vi "temp_FlpLib PI_Controller.vi"(0 "error":sgl format="%#_13g", 1 "reset? (F)":bool, 5 "enable bumpless transfer? (F)":bool, 7 "manual control":T5, 11 "state in":T2, 12 "gains":T3 {"proportional gain" step=0.125}, 13 "output range":T4={"output high (Inf)"=inf, "output low (-Inf)"=-inf}) -> (4 "output":sgl, 6 "error":sgl, 8 "actions":T1, 15 "state out":T2)   [LabVIEW 2016]
uses:
  <vilib>/rvi/Analysis/control/PID/Typedef/niFpgaPID_ManualControl.ctl
  <vilib>/rvi/Analysis/control/PID/Typedef/niFpgaPID_OutputRange.ctl
  <vilib>/rvi/Analysis/control/PID/Typedef/niFpgaPID_PIGains.ctl
  <vilib>/rvi/Analysis/control/PID/Typedef/niFpgaPID_PIState.ctl
  <vilib>/rvi/Analysis/control/PID/Typedef/niFpgaPID_PIActions.ctl
  <userlib>/_NI FLP Library/FPGA/outsideSCTL/FlpLib Multiply Shared Instance 0.vi
  <userlib>/_NI FLP Library/FPGA/outsideSCTL/FlpLib Add Shared Instance 0.vi
  <userlib>/_NI FLP Library/FPGA/outsideSCTL/FlpLib Subtract Shared Instance 0.vi
  <userlib>/_NI FLP Library/FPGA/outsideSCTL/FlpLib In Range and Coerce Shared Instance 0.vi
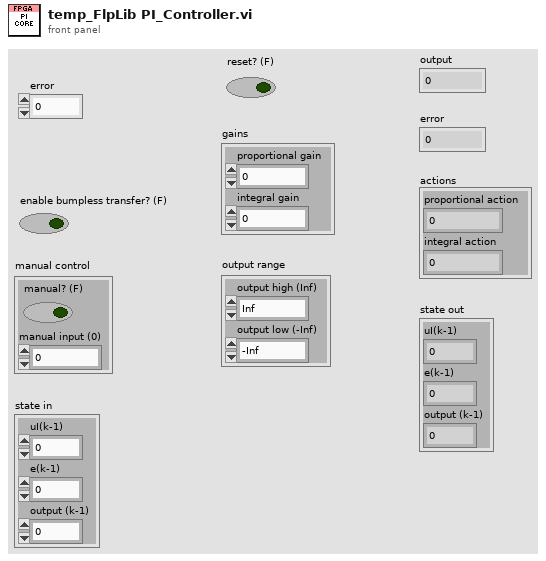
[diagram p1: front panel]
types:
  T1 = typedef "niFpgaPID_PIActions.ctl" = cluster{"proportional action":sgl, "integral action":sgl}
  T2 = typedef "niFpgaPID_PIState.ctl" = cluster{"uI(k-1)":sgl, "e(k-1)":sgl, "output (k-1)":sgl}
  T3 = typedef "niFpgaPID_PIGains.ctl" = cluster{"proportional gain":sgl, "integral gain":sgl}
  T4 = typedef "niFpgaPID_OutputRange.ctl" = cluster{"output high (Inf)":sgl, "output low (-Inf)":sgl}
  T5 = typedef "niFpgaPID_ManualControl.ctl" = cluster{"manual? (F)":bool, "manual input (0)":sgl}
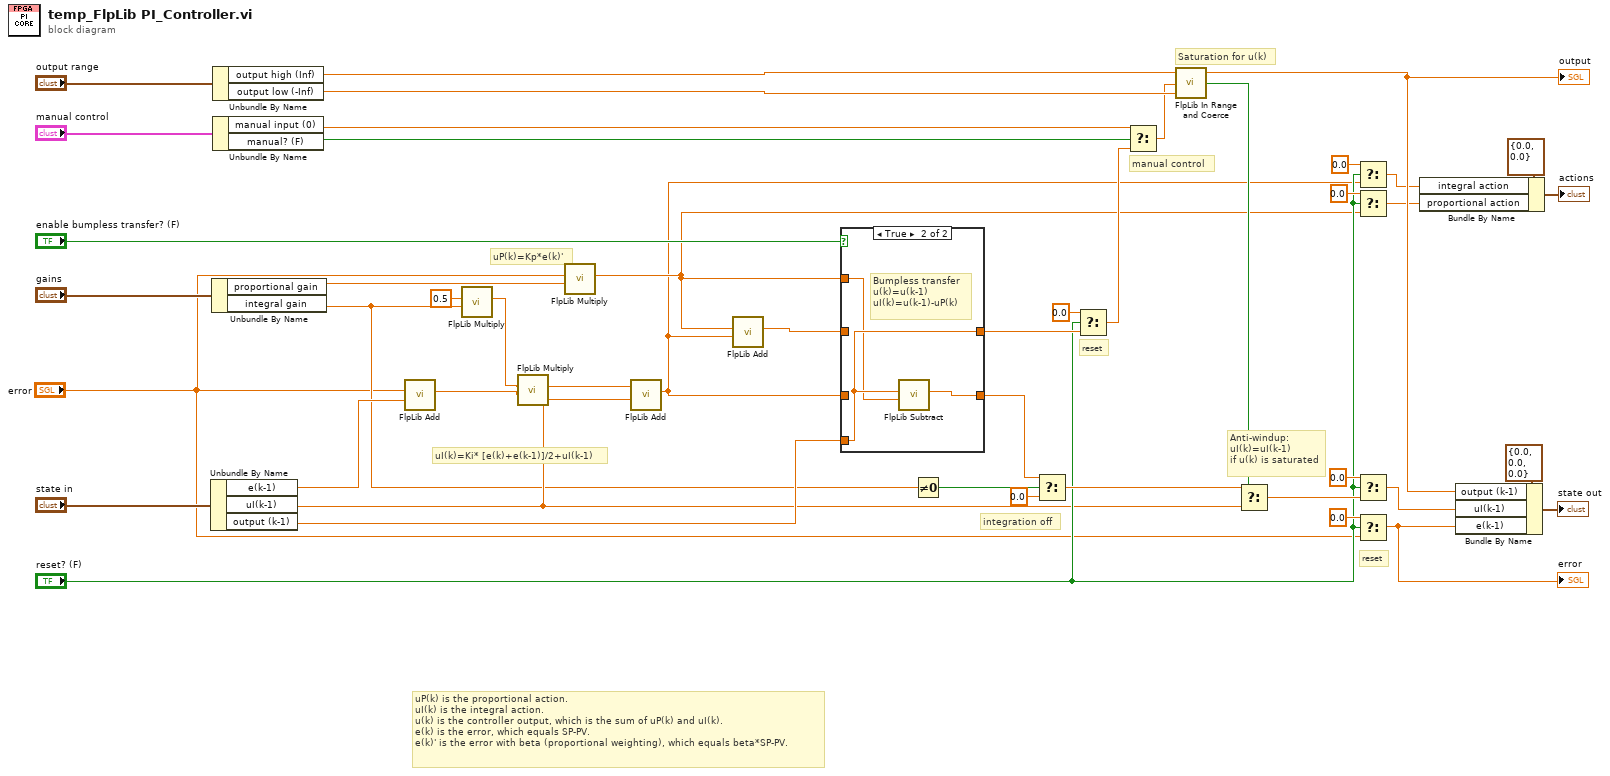
[diagram p0: block diagram]
diagram:
  # "uP(k) is the proportional action.\nuI(k) is the integral action.\nu(k) is the controller output, which is the sum of uP(k) and uI(k).\ne(k) is the error, which equals SP-PV.\ne(k)' is the error with beta (proportional weighting), which equals beta*SP-PV."
  # "integration off"
  # "reset"
  # "manual control"
  # "reset"
  # "Anti-windup:\nuI(k)=uI(k-1) \nif u(k) is saturated"
  # "Saturation for u(k)"
  # "uI(k)=Ki* [e(k)+e(k-1)]/2+uI(k-1)"
  # "uP(k)=Kp*e(k)'"
  n1 = Unbundle By Name("state in") -> ("e(k-1)"=w12:sgl, "uI(k-1)"=w11:sgl, "output (k-1)"=w39:sgl)
  n2 = Unbundle By Name("gains") -> ("proportional gain"=w8:sgl, "integral gain"=w3:sgl)
  n3 = Unbundle By Name("output range") -> ("output high (Inf)"=w27:sgl, "output low (-Inf)"=w26:sgl)
  n4 = Unbundle By Name("manual control") -> ("manual input (0)"=w36:sgl, "manual? (F)"=w35:bool)
  n5 = call-poly <userlib>:"FlpLib Add.vi"("y"=w12, "x"="error") -> ("x+y"=w10:sgl)  [unwired: 5 in]
  n6 = call-poly <userlib>:"FlpLib Multiply.vi"("y"=w3, "x"=sgl 0.5) -> ("x*y"=w4:sgl)  [unwired: 5 in]
  n7 = call-poly <userlib>:"FlpLib Multiply.vi"("y"=w10, "x"=w4) -> ("x*y"=w9:sgl)  [unwired: 5 in]
  n8 = call-poly <userlib>:"FlpLib Multiply.vi"("y"=w8, "x"="error") -> ("x*y"=w7:sgl)  [unwired: 5 in]
  n9 = call-poly <userlib>:"FlpLib Add.vi"("y"=w11, "x"=w9) -> ("x+y"=w6:sgl)  [unwired: 5 in]
  n10 = call-poly <userlib>:"FlpLib Add.vi"("y"=w6, "x"=w7) -> ("x+y"=w5:sgl)  [unwired: 5 in]
  n11 = case shown="True" "enable bumpless transfer? (F)" {
    tunnel: w5 -> [w48 _]
    tunnel: [w48 w51] -> w32
    tunnel: w6 -> [w47 _]
    tunnel: [w47 w49] -> w34
    tunnel: w7 -> [_ w50]
    tunnel: w39 -> [_ w51]
    frame False {
    }
    frame True {
      # "Bumpless transfer\nu(k)=u(k-1)\nuI(k)=u(k-1)-uP(k)"
      n12 = call-poly <userlib>:"FlpLib Subtract.vi"("y"=w50, "x"=w51) -> ("x-y"=w49:sgl)  [unwired: 5 in]
    }
  }
  n13 = Not Equal To 0?(x=w3) -> (x != 0?=w38:bool)
  n14 = Select(t=w34, s=w38, f=sgl 0.0) -> (s? t:f=w16:sgl)
  n15 = Select(t=sgl 0.0 ("f"), s="reset? (F)", f=w32) -> (s? t:f=w31:sgl)
  n16 = Select(t=w36, s=w35, f=w31) -> (s? t:f=w25:sgl)
  n17 = call-poly <userlib>:"FlpLib In Range and Coerce.vi"("lower limit"=w26, "x"=w25, "upper limit"=w27) -> ("in range?"=w28:bool, "coerced(x)"=w24:sgl)  [unwired: 1 in]
  "output" <- w24
  n18 = Select(t=w16, s=w28, f=w11) -> (s? t:f=w17:sgl)
  n19 = Select(t=sgl 0.0, s="reset? (F)", f=w6) -> (s? t:f=w20:sgl)
  n20 = Select(t=sgl 0.0, s="reset? (F)", f=w7) -> (s? t:f=w21:sgl)
  n21 = Select(t=sgl 0.0, s="reset? (F)", f=w17) -> (s? t:f=w15:sgl)
  n22 = Select(t=sgl 0.0, s="reset? (F)", f="error") -> (s? t:f=w13:sgl)
  "error" <- w13
  n23 = Bundle By Name(cluster=T1 {"proportional action"=0.0, "integral action"=0.0} ("actions"), "integral action"=w20, "proportional action"=w21) -> (→"actions":T1)
  n24 = Bundle By Name(cluster=T2 {"uI(k-1)"=0.0, "e(k-1)"=0.0, "output (k-1)"=0.0} ("state out"), "output (k-1)"=w24, "uI(k-1)"=w15, "e(k-1)"=w13) -> (→"state out":T2)
